vi "Progress Bar Example with Process Error.vi"() -> ()   [LabVIEW 2015]
doc: "This example VI illustrates how to implement the process errors handling."
uses:
  Library/New Job Status.vi
  Library/New Item Status.vi
  Library/Class/Error.vi
  Library/Class/Finish.vi
  Library/Simple Progress Bar.lvlib
  Library/Class/Bar.lvclass
panel:
  out "Process Error":errorcluster
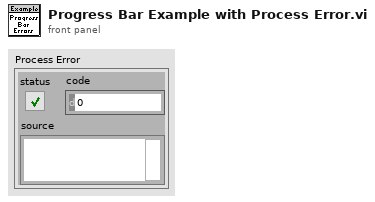
[diagram p1: front panel]
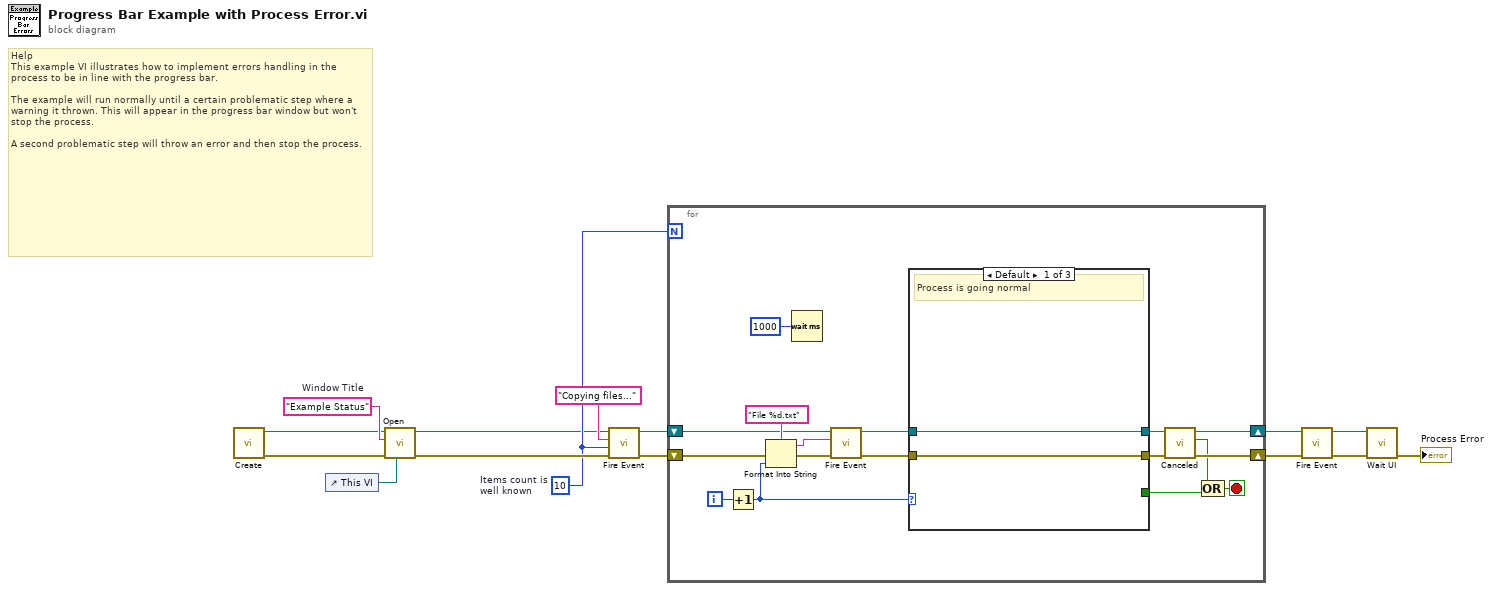
[diagram p0: block diagram]
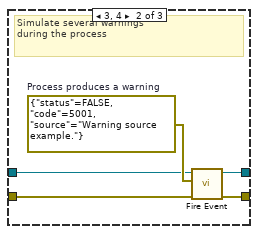
[diagram p2: hidden frame]
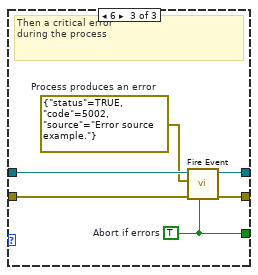
[diagram p3: hidden frame]
diagram:
  w8 = 10  # Items count is  well known
  w14 = "Example Status"  # Window Title
  # "Help\nThis example VI illustrates how to implement errors handling in the process to be in line with the progress bar.\n\nThe example will run normally until a certain problematic step where a warning it thrown. This will appear in the progress bar window but won't stop the process.\n\nA second problematic step will throw an error and then stop the process."
  n1 = call "Create.vi"() -> ("error out"=w15:errorcluster, "Bar out"=w3:refnum<class "Bar.lvclass">)  [unwired: 10 in]
  n2 = control-ref of="This VI"() -> (w4:refnum<vi>)
  n3 = call "Open.vi"("Caller VI"=w4, "error in (no error)"=w15, "Window Title"=w14, "Bar in"=w3) -> ("error out"=w13:errorcluster, "Bar out"=w2:refnum<class "Bar.lvclass">)  [unwired: 6 in]
  n4 = call-poly "Fire Event.vi"("error in (no error)"=w13, "Items Count (unknown)"=w8, "Status"="Copying files...", "Bar in"=w2) -> ("error out"=w9:errorcluster, "Bar out"=w10:refnum<class "Bar.lvclass">)  [unwired: 6 in]
  n5 = for {
    N: w8 -> [_]
    shift-right: [w21] -> w12
    shift-left: w9 -> [w32]
    shift-right: [w16] -> w11
    shift-left: w10 -> [w27]
    i -> [w31]
    stop <- w19 stop-if-true
    n6 = Increment(x=w31) -> (x+1=w25:i32)
    n7 = Format Into String(format string="File %d.txt", error in=w32, w25) -> (resulting string=w26:string, error out=w28:errorcluster)  [unwired: 1 in]
    n8 = Wait (ms)(milliseconds to wait=u32 1000) -> ()  [unwired: 1 out]
    n9 = call-poly "Fire Event.vi"("error in (no error)"=w28, "Status"=w26, "Bar in"=w27) -> ("error out"=w24:errorcluster, "Bar out"=w22:refnum<class "Bar.lvclass">)  [unwired: 7 in]
    n10 = case shown="Default" w25 {
      tunnel: w24 -> [w34 w38 w43]
      tunnel: [w34 w35 w42] -> w23
      tunnel: [w33 w36 w44] -> w17
      tunnel: w22 -> [w33 w37 w45]
      tunnel: [_ _ w40] -> w18
      frame Default {
        # "Process is going normal"
      }
      frame 3, 4 {
        w39 = errorcluster {"status"=FALSE, "code"=5001, "source"="Warning source example."}  # Process produces a warning
        # "Simulate several warnings \nduring the process"
        n11 = call-poly "Fire Event.vi"("error in (no error)"=w38, "Process Error"=w39, "Bar in"=w37) -> ("error out"=w35:errorcluster, "Bar out"=w36:refnum<class "Bar.lvclass">)  [unwired: 7 in]
      }
      frame 6 {
        w40 = TRUE  # Abort if errors
        w41 = errorcluster {"status"=TRUE, "code"=5002, "source"="Error source example."}  # Process produces an error
        # "Then a critical error \nduring the process"
        n12 = call-poly "Fire Event.vi"("Abort if errors"=w40, "error in (no error)"=w43, "Process Error"=w41, "Bar in"=w45) -> ("error out"=w42:errorcluster, "Bar out"=w44:refnum<class "Bar.lvclass">)  [unwired: 6 in]
      }
    }
    n13 = call "Canceled.vi"("error in (no error)"=w23, "Bar in"=w17) -> ("error out"=w21:errorcluster, "Canceled by user?"=w20:bool, "Bar out"=w16:refnum<class "Bar.lvclass">)  [unwired: 7 in]
    n14 = Compound Arithmetic op=OR(w20, w18) -> (w19:bool)
  }
  n15 = call-poly "Fire Event.vi"("error in (no error)"=w12, "Bar in"=w11) -> ("error out"=w6:errorcluster, "Bar out"=w1:refnum<class "Bar.lvclass">)  [unwired: 8 in]
  n16 = call "Wait UI.vi"("error in (no error)"=w6, "Bar in"=w1) -> ("error out"=→"Process Error":errorcluster)  [unwired: 6 in, 3 out]
